vi "ctet_dio_User Main.vi"() -> ()   [LabVIEW 2019, in "ctet_dio_User Library.lvlib"]
uses:
  ctet_dio_User Library.lvlib
  Servers/ctet_dio/ctet_dio Class/typeDefs/Server State Data.ctl
  Types/DIOSessions.ctl
  Types/DISession.ctl
  Types/DOSession.ctl
  Types/StreamReadDI.ctl
  Servers/ctet_dio/gRPC lvSupport/Server API/typeDefs/grpcId.ctl
  Servers/ctet_dio/ctet_dio Class/ctet_dio.lvclass/ctet_dio.ctl
  Servers/ctet_dio/ctet_dio Class/ctet_dio.lvclass
  Servers/ctet_dio/gRPC lvSupport/gprc-lvsupport.lvlib
panel:
  in  "Stop":bool
  in  "Server Address":string="0.0.0.0:50054"
  in  "Server Certificate File (.crt)":path
  in  "Server Key File (.key)":path
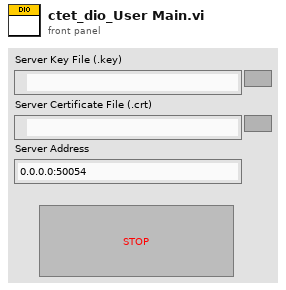
[diagram p1: front panel]
types:
  T1 = typedef "ctet_dio_User Library.lvlib/DIOSessions.ctl" = cluster{"Array of DI Sessions":T2[], "Array of DO Sessions":T3[], "Stream ReadDI":T4}
  T2 = typedef "ctet_dio_User Library.lvlib/DISession.ctl" = cluster{"DI Task":refnum<k21>, "DISessionName":string}
  T3 = typedef "ctet_dio_User Library.lvlib/DOSession.ctl" = cluster{"DO Task":refnum<k21>, "DOSessionName":string}
  T4 = typedef "ctet_dio_User Library.lvlib/StreamReadDI.ctl" = cluster{"gRPCid ReadDI":T5, "DISessionName":string, "Stream Status ReadDI":bool, "Async Stop ReadDI Queue":refnum<queue>, "DI Task":refnum<k21>, "ms to wait":u32}
  T5 = typedef "ctet_dio.lvlib/gprc-lvsupport.lvlib/grpcId.ctl" = u64
  T6 = typedef "ctet_dio.lvlib/ctet_dio.lvclass/Server State Data.ctl" = cluster{"Data":string}
  T7 = typedef "ctet_dio.lvlib/ctet_dio.lvclass/Server gRPC UEs.ctl" = cluster{"Invoke gRPC UE":refnum<user-event>, "Query gRPC UE":refnum<user-event>, "Register gRPC UE":refnum<user-event>, "OpenDISession gRPC UE":refnum<user-event>, "OpenDOSession gRPC UE":refnum<user-event>, "ReadDI gRPC UE":refnum<user-event>, "StopDI gRPC UE":refnum<user-event>, "WriteDO gRPC UE":refnum<user-event>, "CloseDISession gRPC UE":refnum<user-event>, "CloseDOSession gRPC UE":refnum<user-event>}
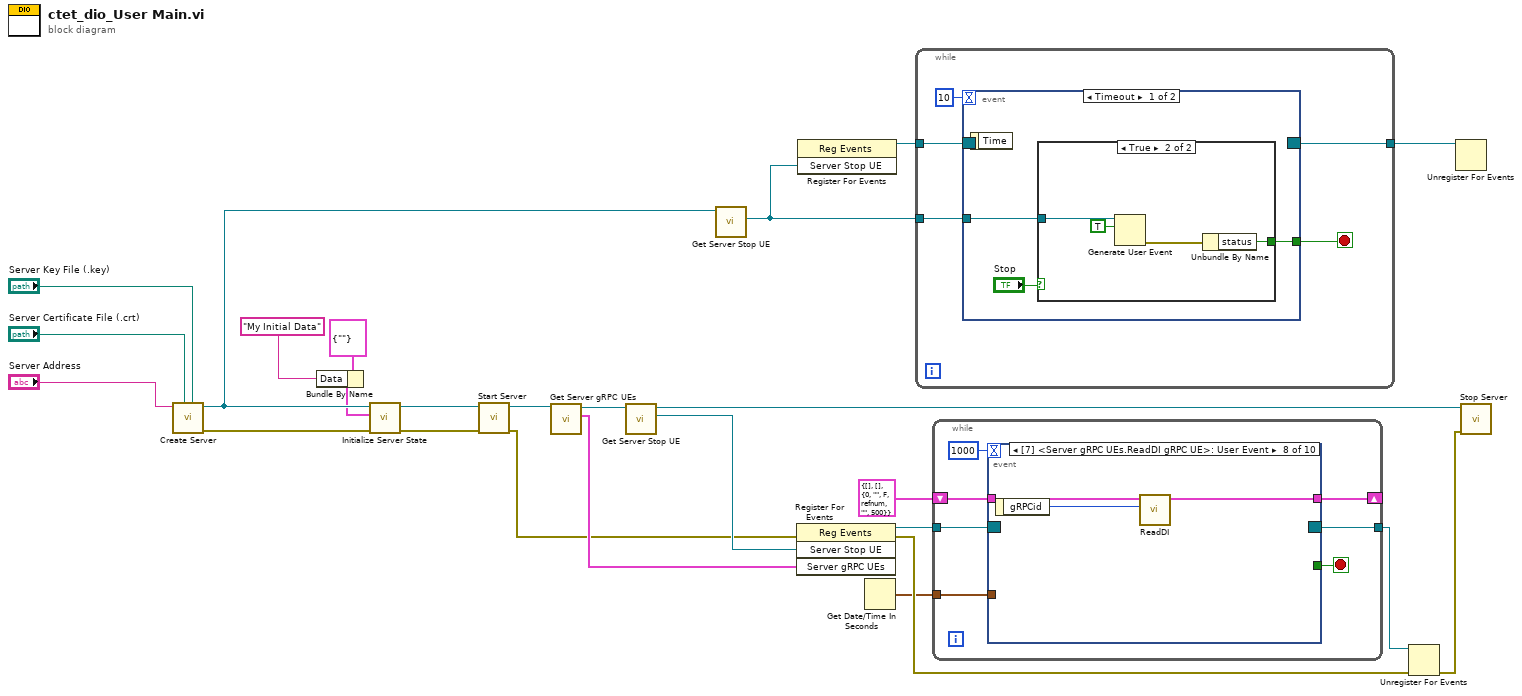
[diagram p0: block diagram]
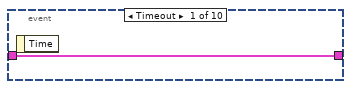
[diagram p2: hidden frame]
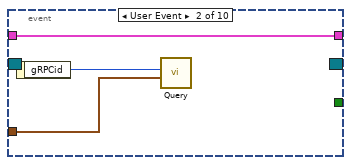
[diagram p3: hidden frame]
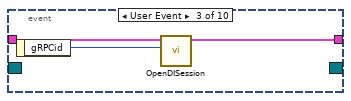
[diagram p4: hidden frame]
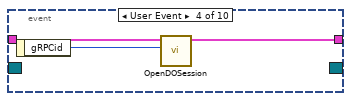
[diagram p5: hidden frame]
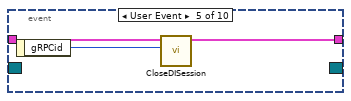
[diagram p6: hidden frame]
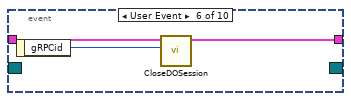
[diagram p7: hidden frame]
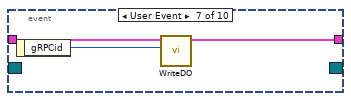
[diagram p8: hidden frame]
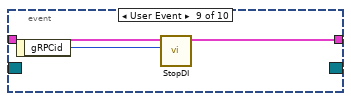
[diagram p9: hidden frame]
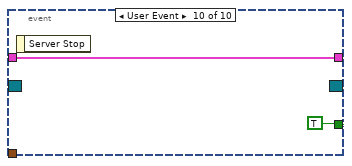
[diagram p10: hidden frame]
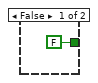
[diagram p11: hidden frame]
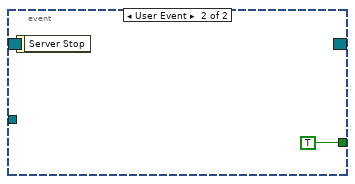
[diagram p12: hidden frame]
diagram:
  n1 = call "Create Server.vi"("Server Key File (.key)"="Server Key File (.key)", "Server Certificate File (.crt)"="Server Certificate File (.crt)", "Server Address"="Server Address") -> ("error out"=w19:errorcluster, "gRPC Server out"=w16:refnum<class "ctet_dio.lvclass">)  [unwired: 7 in]
  n2 = Bundle By Name(cluster=T6 {"Data"=""} ("Initial State"), "Data"="My Initial Data") -> (w14:T6)
  n3 = call "Initialize Server State.vi"("error in (no error)"=w19, "Initial State"=w14, "gRPC Server in"=w16) -> ("error out"=w18:errorcluster, "gRPC Server out"=w17:refnum<class "ctet_dio.lvclass">)  [unwired: 7 in]
  n4 = call "Start Server.vi"("error in (no error)"=w18, "gRPC Server in"=w17) -> ("error out"=w6:errorcluster, "gRPC Server out"=w7:refnum<class "ctet_dio.lvclass">)  [unwired: 8 in]
  n5 = call "Get Server gRPC UEs.vi"("OOP Server in"=w7) -> ("Server gRPC UEs"=w10:T7, "OOP Server out"=w12:refnum<class "ctet_dio.lvclass">)  [unwired: 9 in]
  n6 = call "Get Server Stop UE.vi"("OOP Server in"=w12) -> ("Server Stop UE"=w11:refnum<user-event>, "OOP Server out"=w4:refnum<class "ctet_dio.lvclass">)  [unwired: 9 in]
  n7 = call "Get Server Stop UE.vi"("OOP Server in"=w16) -> ("Server Stop UE"=w20:refnum<user-event>)  [unwired: 9 in, 1 out]
  n8 = register-events(error in=w6, w11, w10) -> (reference out=w9:refnum<event-registration>, error out=w5:errorcluster)  [unwired: 1 in]
  n9 = register-events(w20) -> (reference out=w22:refnum<event-registration>)  [unwired: 2 in, 1 out]
  n10 = Get Date/Time In Seconds() -> (seconds since 1Jan1904=w2:timestamp)
  n11 = while {
    tunnel: w20 -> [w30]
    tunnel: w22 -> [w29]
    tunnel: [w27] -> w21
    stop <- w28 stop-if-true
    n12 = event shown="[0] Timeout" {
      selector: w29 -> [_ _]
      dyn-events: [_ _] -> w27
      timeout: 10 -> [_ _]
      tunnel: w30 -> [w32 _]
      tunnel: [w33 TRUE] -> w28
      event Timeout {
        n13 = event-data() -> ()  [unwired: 1 in, 1 out]
        n14 = case shown="True" "Stop" {
          tunnel: [FALSE ("status") w36] -> w33
          tunnel: w32 -> [_ w35]
          frame False {
          }
          frame True {
            n15 = Generate User Event(user event=w35, event data cluster=TRUE ("event data")) -> (error out=w37:errorcluster)  [unwired: 2 in, 1 out]
            n16 = Unbundle By Name(w37) -> ("status"=w36:bool)
          }
        }
      }
      event User Event {
        n17 = event-data() -> ()  [unwired: 1 in, 1 out]
      }
    }
  }
  n18 = while {
    tunnel: w9 -> [w46]
    tunnel: [w44] -> w8
    tunnel: w2 -> [w42]
    shift-right: [w40] -> _
    shift-left: T1 {"Array of DI Sessions"=[], "Array of DO Sessions"=[], "Stream ReadDI"={"gRPCid ReadDI"=0, "DISessionName"="", "Stream Status ReadDI"=FALSE, "Async Stop ReadDI Queue"=refnum, "DI Task"="", "ms to wait"=500}} ("DIOSessions") -> [w41]
    stop <- w45 stop-if-true
    n19 = event "RPC Methods Event Structure" shown="[7] <Server gRPC UEs.ReadDI gRPC UE>: User Event" {
      selector: w46 -> [_ _ _ _ _ _ _ _ _ _]
      dyn-events: [_ _ _ _ _ _ _ _ _ _] -> w44
      timeout: 1000 -> [_ _ _ _ _ _ _ _ _ _]
      tunnel: [_ _ _ _ _ _ _ _ _ TRUE] -> w45
      tunnel: w42 -> [_ w49 _ _ _ _ _ _ _ _]
      tunnel: w41 -> [w47 w48 w52 w55 w58 w61 w64 w67 w70 w72]
      tunnel: [w47 w48 w51 w54 w57 w60 w63 w66 w69 w72] -> w40
      event Timeout {
        n20 = event-data() -> ()  [unwired: 1 in, 1 out]
      }
      event User Event {
        n21 = event-data() -> ("gRPCid"=w50:T5)  [unwired: 1 in]
        n22 = call "Query.vi"("current time"=w49, "gRPCid"=w50) -> ()  [unwired: 9 in, 1 out]
      }
      event User Event {
        n23 = event-data() -> ("gRPCid"=w53:T5)  [unwired: 1 in]
        n24 = call "OpenDISession.vi"("gRPCid"=w53, "DIOSessions In"=w52) -> ("DIOSessions Out"=w51:T1)  [unwired: 8 in, 1 out]
      }
      event User Event {
        n25 = event-data() -> ("gRPCid"=w56:T5)  [unwired: 1 in]
        n26 = call "OpenDOSession.vi"("gRPCid"=w56, "DIOSessions In"=w55) -> ("DIOSessions Out"=w54:T1)  [unwired: 8 in, 1 out]
      }
      event User Event {
        n27 = event-data() -> ("gRPCid"=w59:T5)  [unwired: 1 in]
        n28 = call "CloseDISession.vi"("gRPCid"=w59, "DIOSessions In"=w58) -> ("DIOSessions Out"=w57:T1)  [unwired: 8 in, 1 out]
      }
      event User Event {
        n29 = event-data() -> ("gRPCid"=w62:T5)  [unwired: 1 in]
        n30 = call "CloseDOSession.vi"("gRPCid"=w62, "DIOSessions In"=w61) -> ("DIOSessions Out"=w60:T1)  [unwired: 8 in, 1 out]
      }
      event User Event {
        n31 = event-data() -> ("gRPCid"=w65:T5)  [unwired: 1 in]
        n32 = call "WriteDO.vi"("gRPCid"=w65, "DIOSessions In"=w64) -> ("DIOSessions Out"=w63:T1)  [unwired: 8 in, 1 out]
      }
      event User Event {
        n33 = event-data() -> ("gRPCid"=w68:T5)  [unwired: 1 in]
        n34 = call "ReadDI.vi"("gRPCid"=w68, "DIOSessions In"=w67) -> ("DIOSessions Out"=w66:T1)  [unwired: 8 in, 1 out]
      }
      event User Event {
        n35 = event-data() -> ("gRPCid"=w71:T5)  [unwired: 1 in]
        n36 = call "StopDI.vi"("gRPCid"=w71, "DIOSessions In"=w70) -> ("DIOSessions Out"=w69:T1)  [unwired: 8 in, 1 out]
      }
      event User Event {
        n37 = event-data() -> ()  [unwired: 1 in, 1 out]
      }
    }
  }
  n38 = Unregister For Events(event registration refnum=w8, error in=w5) -> (error out=w3:errorcluster)
  n39 = Unregister For Events(event registration refnum=w21) -> ()  [unwired: 1 in, 1 out]
  n40 = call "Stop Server.vi"("error in (no error)"=w3, "gRPC Server in"=w4) -> ()  [unwired: 9 in, 1 out]
